vi "DoubleClick.vi"(7 "Fill Color":T7=16860, 8 "error in (no error)":errorcluster, 9 "Data in":T1={"Class"={"Ants"=refnum, "Layer"=refnum, "Templates"=refnum, "Icon"=refnum, "Glyph"=refnum, "Settings"=refnum, "Tools"=refnum}, "Ref"={"Add Layer"=refnum, "Remove Layer"=refnum, "Line Text"=[], "Body Text Spec"=refnum, "DNL_Font"=refnum, "glyph path str"=refnum, "templates path str"=refnum, "Arrow Up"=refnum, "Arrow Down"=refnum, "IE VI Ref"=refnum, "Glyphs tree"=refnum, "Templates tree"=refnum, "Layer Icon Text"=refnum, "Layer Template"=refnum, "Body Text"=refnum, "Search Templates"=refnum, "TextMarker"=refnum, "Tab Control"=refnum, "Search Glyphs"=refnum, "Line Color"=refnum, "DNL_Glyphs []"=refnum, "Fill Color"=refnum, "Tools"=refnum, "Icon"=refnum, "Preview"=refnum, "Ants"=refnum, "Terminals"=refnum, "menu reference"=refnum, "LayerNames"=[], "GlyphLoadAnimation"=refnum, "TemplateLoadAnimation"=refnum, "refreshGlyphs"=refnum, "refreshTemplates"=refnum}, "Support"={"AntsRect"={"left"=0, "top"=0, "right"=0, "bottom"=0}, "Mouse Move Coords"={"Horizontal"=0, "Vertical"=0}, "Mouse Down Coords"={"Horizontal"=0, "Vertical"=0}, "Temp Coord"={"Horizontal"=0, "Vertical"=0}, "Action"=enum."Default", "Edge Color"=4914962, "Fill Color"=16860, "Mouse Down?"=FALSE, "Draft Mode?"=FALSE, "Temp Icon"=bytes[3102], "CTRL Pressed"=FALSE, "Move Selection?"=FALSE, "AntsRect Orig"={"left"=0, "top"=0, "right"=0, "bottom"=0}, "Text"="", "TM Set?"=FALSE, "Mouse inside icon?"=FALSE, "Tool (old value)"=0, "Pencil Move Color"=0, "Swap Colors?"=FALSE, "Shift pressed?"=FALSE}}, 10 "Edge Color":T7=16860, 11 "Tools Paint in":refnum<class "Tools Paint.lvclass">) -> (0 "error out":errorcluster, 1 "Name":string, 2 "new picture":picture, 3 "Tools Paint out":refnum<class "Tools Paint.lvclass">, 4 "Active Tool":T8=enum."Ellipse", 5 "Invalid Picture?":bool)   [LabVIEW 2020, in "Tools Paint.lvclass"]
uses:
  Tools Paint.lvclass
  Ants/Ants.lvclass
  FakedArray/FakedArray.lvclass
  vi.lib/LabVIEW Icon API/lv_icon/Classes/Icon/Icon.lvclass
  Icon Library/Glyph.lvclass
  Settings/Settings.lvclass
  Tools Paint.lvclass/Tools Paint.ctl
  vi.lib/LabVIEW Icon API/lv_icon/Controls/IEColor.ctl
  Controls/Circle.ctl
  Controls/Dropper.ctl
  Controls/FCircle.ctl
  Controls/Fill.ctl
  Controls/FRect.ctl
  Controls/Line.ctl
  Controls/Move.ctl
  Controls/Pen.ctl
  Controls/IERect.ctl
  Controls/Rubber.ctl
  Controls/Selection.ctl
  Controls/Text.ctl
  Controls/Tools.ctl
  <vilib>/Utility/miscctls.llb/LVPoint32TypeDef.ctl
  Controls/SupportClass_Action.ctl
  Controls/SupportClass.ctl
  Controls/References Cluster.ctl
  vi.lib/LabVIEW Icon API/lv_icon/lv_icon.lvlib
  Controls/IE Classes.ctl
  Controls/Global Data.ctl
panel:
  in  "String 2":string="Border"
  in  "String":string="Filled"
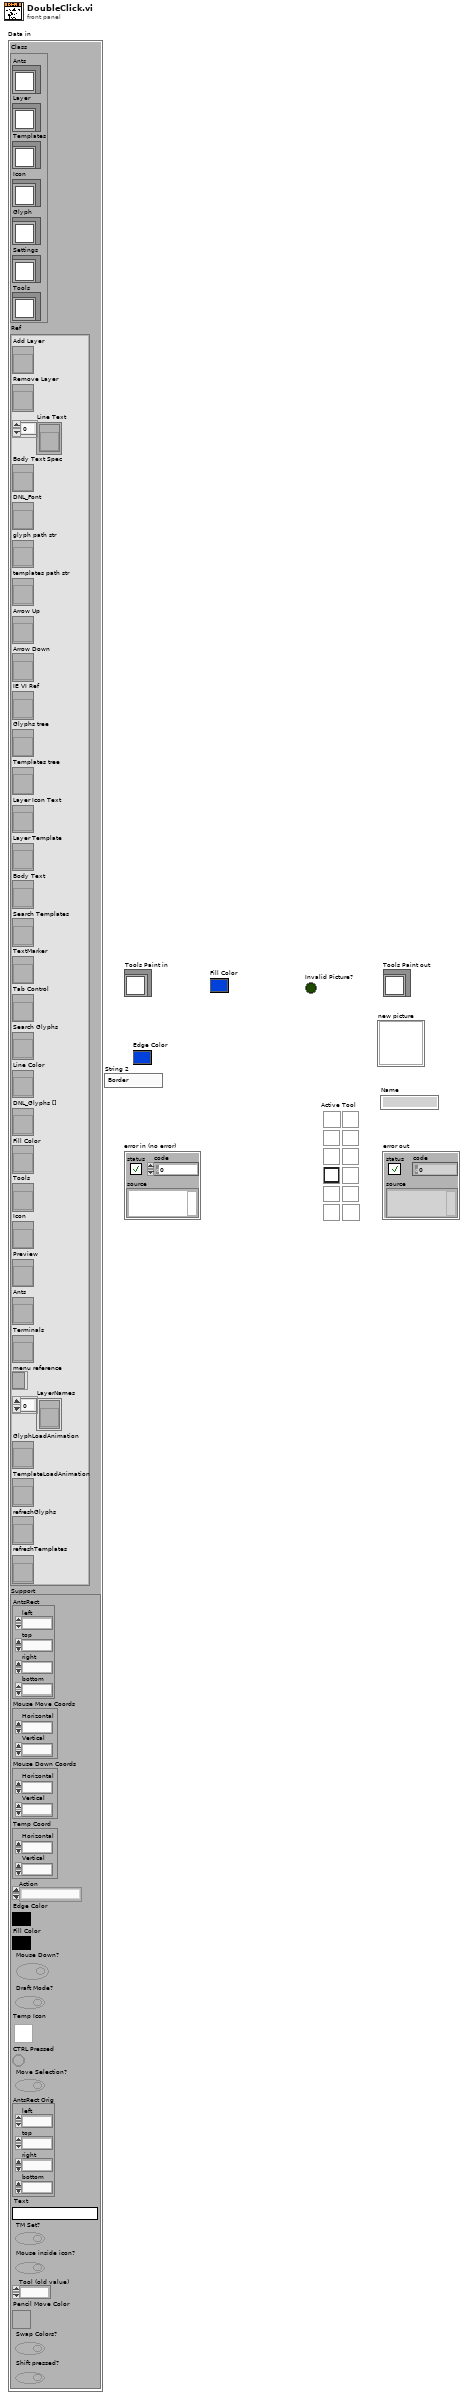
[diagram p1: front panel]
types:
  T1 = typedef "lv_icon.lvlib/Global Data.ctl" = cluster{"Class":T2, "Ref":T3, "Support":T4}
  T2 = typedef "IE Classes.ctl" = cluster{"Ants":refnum<class "Ants.lvclass">, "Layer":refnum<class "FakedArray.lvclass">, "Templates":refnum<class "FakedArray.lvclass">, "Icon":refnum<class "Icon.lvclass">, "Glyph":refnum<class "Glyph.lvclass">, "Settings":refnum<class "Settings.lvclass">, "Tools":refnum<class "Tools Paint.lvclass">}
  T3 = typedef "lv_icon.lvlib/References Cluster.ctl" = cluster{"Add Layer":refnum<vi>, "Remove Layer":refnum<vi>, "Line Text":refnum<vi>[], "Body Text Spec":refnum<vi>, "DNL_Font":refnum<vi>, "glyph path str":refnum<vi>, "templates path str":refnum<vi>, "Arrow Up":refnum<vi>, "Arrow Down":refnum<vi>, "IE VI Ref":refnum<vi>, "Glyphs tree":refnum<vi>, "Templates tree":refnum<vi>, "Layer Icon Text":refnum<vi>, "Layer Template":refnum<vi>, "Body Text":refnum<vi>, "Search Templates":refnum<vi>, "TextMarker":refnum<vi>, "Tab Control":refnum<vi>, "Search Glyphs":refnum<vi>, "Line Color":refnum<vi>, "DNL_Glyphs []":refnum<vi>, "Fill Color":refnum<vi>, "Tools":refnum<vi>, "Icon":refnum<vi>, "Preview":refnum<vi>, "Ants":refnum<vi>, "Terminals":refnum<vi>, "menu reference":refnum<k9>, "LayerNames":refnum<vi>[], "GlyphLoadAnimation":refnum<vi>, "TemplateLoadAnimation":refnum<vi>, "refreshGlyphs":refnum<vi>, "refreshTemplates":refnum<vi>}
  T4 = typedef "SupportClass.ctl" = cluster{"AntsRect":cluster{"left":i16, "top":i16, "right":i16, "bottom":i16}, "Mouse Move Coords":T5, "Mouse Down Coords":T5, "Temp Coord":T5, "Action":T6, "Edge Color":T7, "Fill Color":T7, "Mouse Down?":bool, "Draft Mode?":bool, "Temp Icon":picture, "CTRL Pressed":bool, "Move Selection?":bool, "AntsRect Orig":cluster{"left":i16, "top":i16, "right":i16, "bottom":i16}, "Text":string, "TM Set?":bool, "Mouse inside icon?":bool, "Tool (old value)":u32, "Pencil Move Color":u32, "Swap Colors?":bool, "Shift pressed?":bool}
  T5 = typedef "LVPoint32TypeDef.ctl" = cluster{"Horizontal":i32, "Vertical":i32}
  T6 = typedef "SupportClass_Action.ctl" = enum16{"Default", "Move Selection", "Glyph Library", "Tool"}
  T7 = typedef "IEColor.ctl" = u32
  T8 = typedef "Tools.ctl" = enum32{"Pencil", "Line", "Dropper", "Fill", "Rectangle", "Filled Rectangle", "Ellipse", "Filled Ellipse", "Eraser", "Text", "Select", "Move"}
  T9 = cluster{"left":i16, "top":i16, "right":i16, "bottom":i16}
  T10 = cluster{"Left":i32, "Top":i32, "Right":i32, "Bottom":i32}
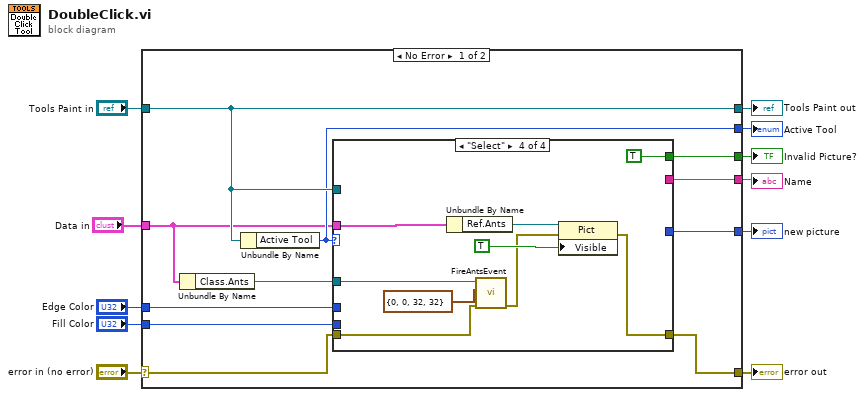
[diagram p0: block diagram]
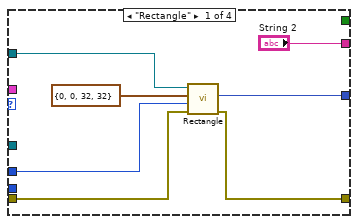
[diagram p2: hidden frame]
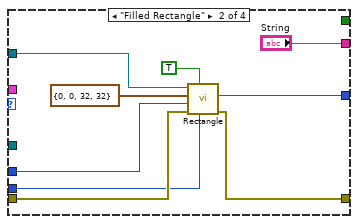
[diagram p3: hidden frame]
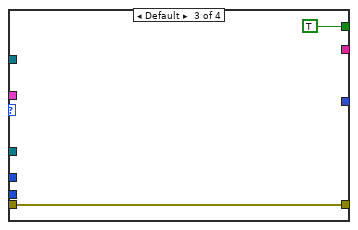
[diagram p4: hidden frame]
diagram:
  n1 = case shown="No Error" "error in (no error)" {
    selector: "error in (no error)" -> [w21 w51]
    tunnel: [w20 w51] -> w10
    tunnel: [w18 w50] -> w8
    tunnel: "Tools Paint in" -> [w18 w50]
    tunnel: "Edge Color" -> [w22 _]
    tunnel: [w19 _] -> w6
    tunnel: [w17 _] -> w5
    tunnel: [w16 _] -> w4
    tunnel: [w15 _] -> w3
    tunnel: "Fill Color" -> [w14 _]
    tunnel: "Data in" -> [w12 _]
    frame No Error {
      n2 = Unbundle By Name(w12) -> ("Class.Ants"=w13:refnum<class "Ants.lvclass">)
      n3 = Unbundle By Name(w18) -> ("Active Tool"=w15:T8)
      n4 = case shown="\"Select\"" w15 {
        tunnel: w22 -> [w28 w37 _ _]
        tunnel: w21 -> [w27 w36 w40 w41]
        tunnel: [w26 w35 w40 w43] -> w20
        tunnel: [w25 w34 _ _] -> w19
        tunnel: w18 -> [w24 w33 _ _]
        tunnel: [_ _ TRUE TRUE] -> w17
        tunnel: ["String 2" "String" _ _] -> w16
        tunnel: w13 -> [_ _ _ w48]
        tunnel: w14 -> [_ w30 _ _]
        tunnel: w12 -> [_ _ _ w42]
        frame "Rectangle" {
          n5 = call-dynamic "Rectangle.vi"("error in (no error)"=w27, "Edge Color"=w28, "rect"=T9 {"left"=0, "top"=0, "right"=32, "bottom"=32}, "Tools Paint in"=w24) -> ("error out"=w26:errorcluster, "new picture"=w25:picture)  [unwired: 2 in, 4 out]
        }
        frame "Filled Rectangle" {
          n6 = call-dynamic "Rectangle.vi"("Fill Color"=w30, "fill?(F)"=TRUE, "error in (no error)"=w36, "Edge Color"=w37, "rect"=T9 {"left"=0, "top"=0, "right"=32, "bottom"=32}, "Tools Paint in"=w33) -> ("error out"=w35:errorcluster, "new picture"=w34:picture)  [unwired: 4 out]
        }
        frame Default {
        }
        frame "Select" {
          n7 = Unbundle By Name(w42) -> ("Ref.Ants"=w46:refnum<vi>)
          n8 = call "FireAntsEvent.vi"("error in (no error)"=w41, "Rectangle (default: deselect)"=T10 {"Left"=0, "Top"=0, "Right"=32, "Bottom"=32} ("Rectangle"), "Ants in"=w48) -> ("error out"=w44:errorcluster)  [unwired: 1 in, 7 out]
          n9 = property class="Pict"(reference=w46, error in=w44, "Visible"=TRUE) -> (error out=w43:errorcluster)  [unwired: 1 out]
        }
      }
    }
    frame Error {
    }
  }
  "error out" <- w10
  "Tools Paint out" <- w8
  "new picture" <- w6
  "Name" <- w4
  "Invalid Picture?" <- w5
  "Active Tool" <- w3
